vi "Test Graph Module API.vi"() -> ()   [LabVIEW 2020]
doc: "Graph Module API Tester."
uses:
  Graph Module.lvlib
panel:
  in  "X Backw":bool
  in  "Y Forw":bool
  in  "Y Backw":bool
  in  "X Forw":bool
  in  "XY Coord":cluster{"X":dbl, "Y":dbl}={"X"=1400.0, "Y"=200.0}
  in  "Mark Coord":bool
  in  "Path":path=path "D:/Git/Graph-Extensions-LabVIEW-master/dxf/#163_CAD2000_.dxf"
  in  "Load DXF":bool
  in  "Run as Singleton?":bool
  in  "Show Block Diagram":bool
  in  "Refresh Modules":bool
  out "Active Modules":string[](array[string])
  in  "Stop Module":bool
  in  "Select Module":i32(ring)=-1 caption="Select Module\nTo send Request to" items=["All"=-1, "1"=1]
  in  "Run New Module":bool
  in  "Hide Module Panel":bool
  in  "Show Module Panel":bool
  out "Status":string
  # "This VI tests the API for the Module."
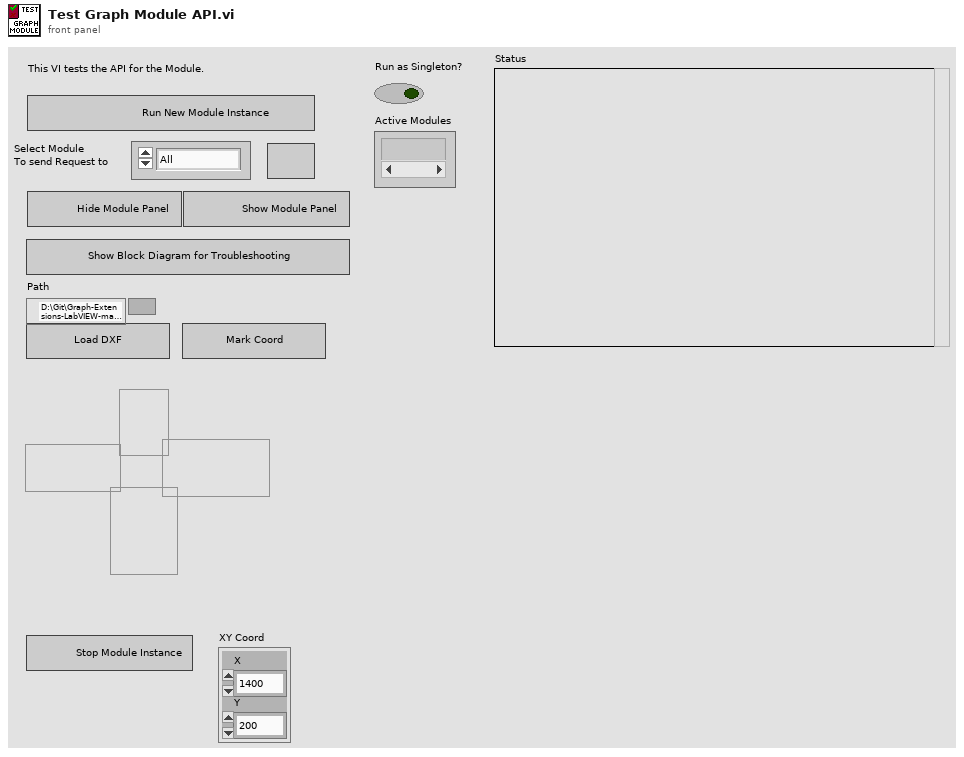
[diagram p1: front panel]
types:
  T1 = typedef "Graph Module.lvlib/Broadcast Events--cluster.ctl" = cluster{"Module Did Init":refnum<user-event>, "Status Updated":refnum<user-event>, "Error Reported":refnum<user-event>, "Module Did Stop":refnum<user-event>, "Update Module Execution Status":refnum<user-event>, "Broadcast Coord":refnum<user-event>}
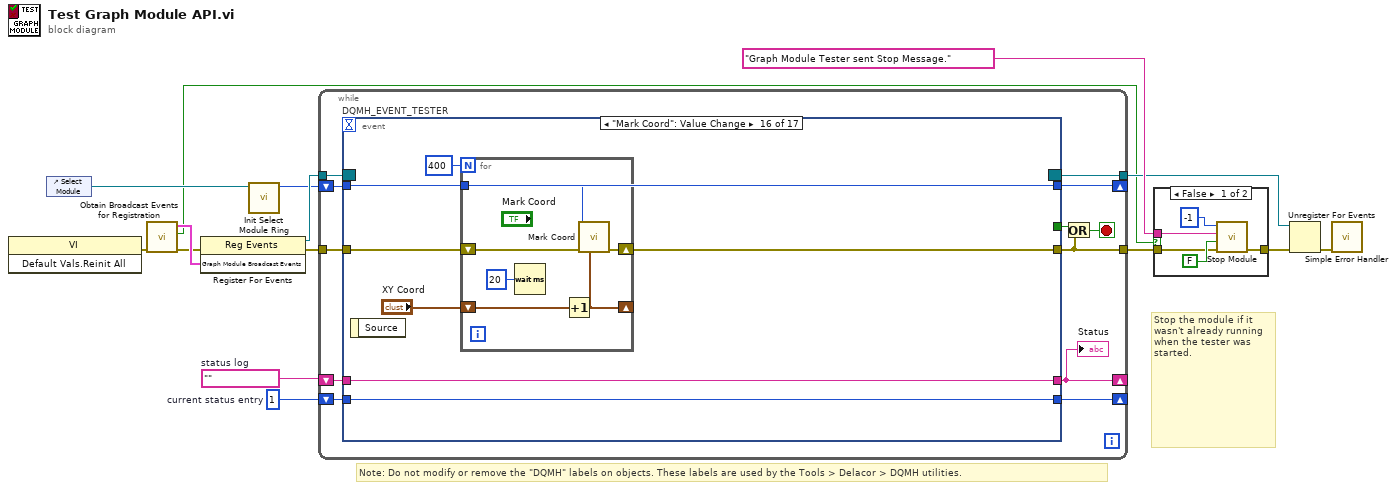
[diagram p0: block diagram]
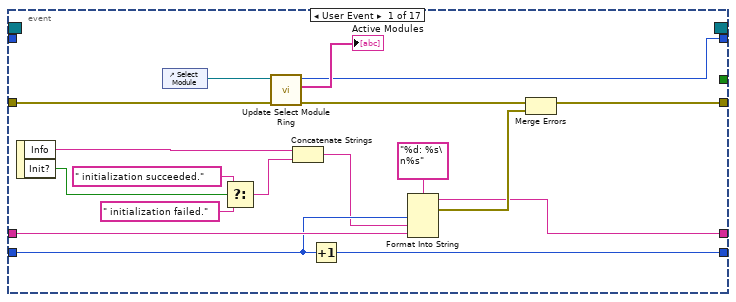
[diagram p3: hidden frame]
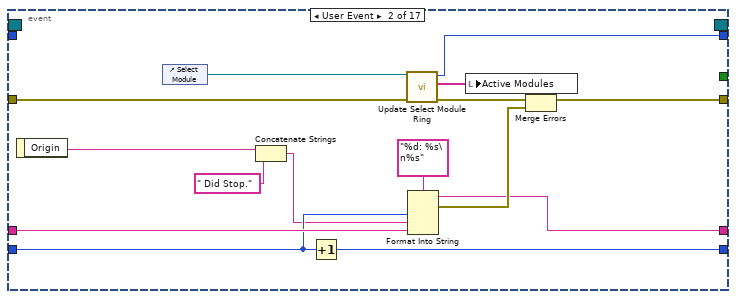
[diagram p4: hidden frame]
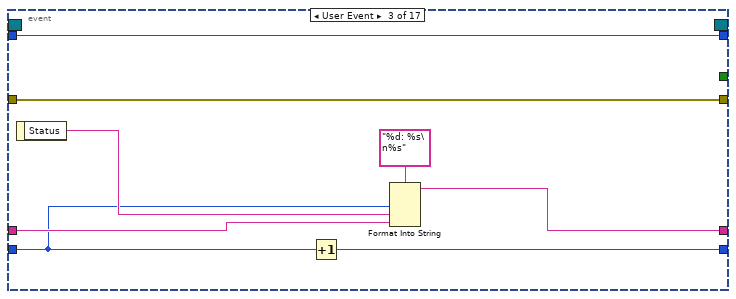
[diagram p5: hidden frame]
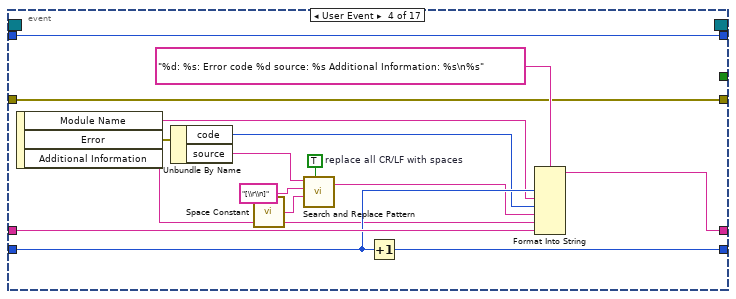
[diagram p6: hidden frame]
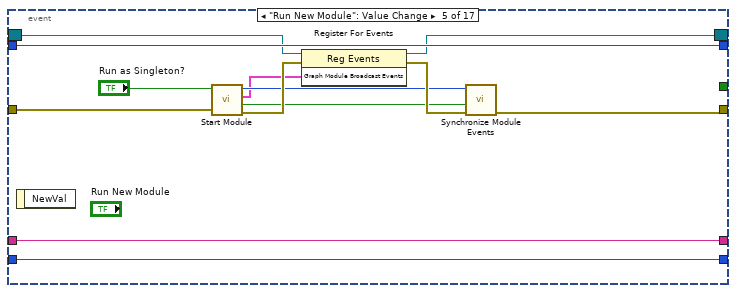
[diagram p7: hidden frame]
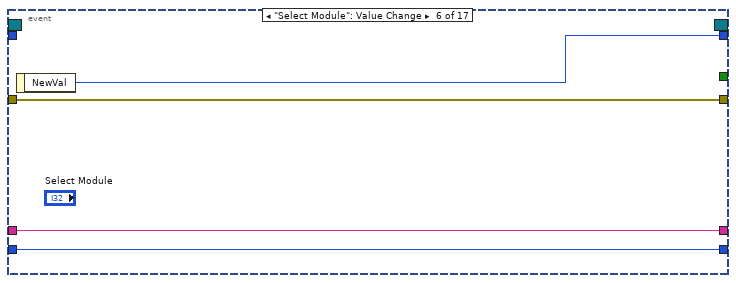
[diagram p8: hidden frame]
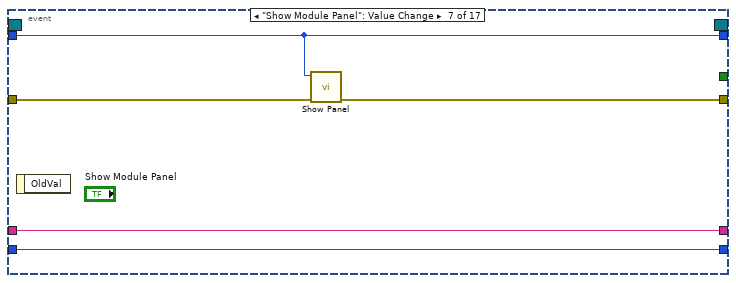
[diagram p9: hidden frame]
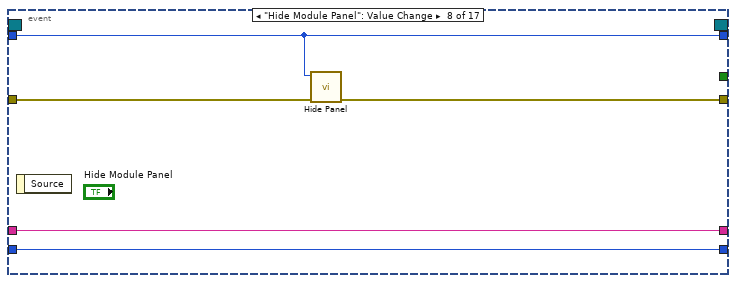
[diagram p10: hidden frame]
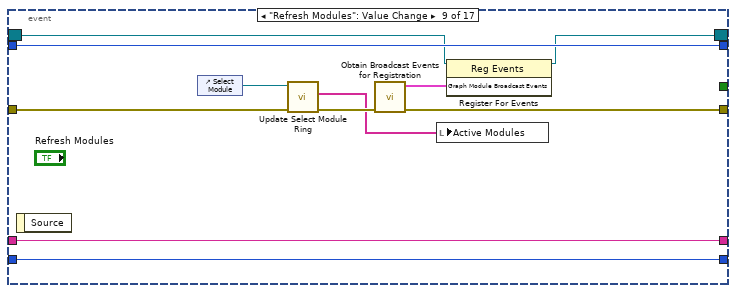
[diagram p11: hidden frame]
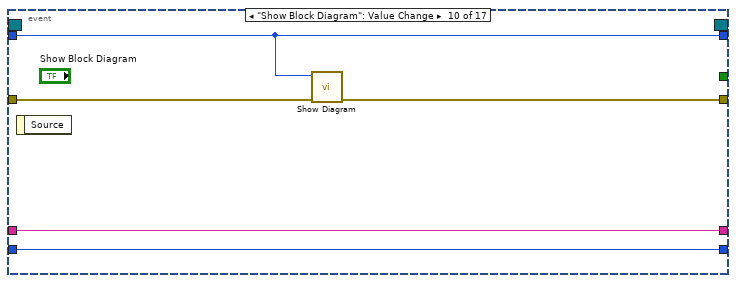
[diagram p12: hidden frame]
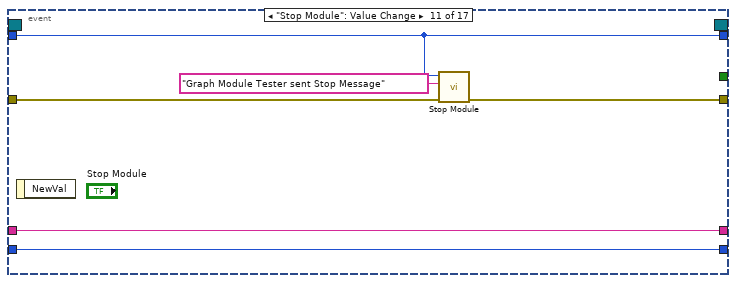
[diagram p13: hidden frame]
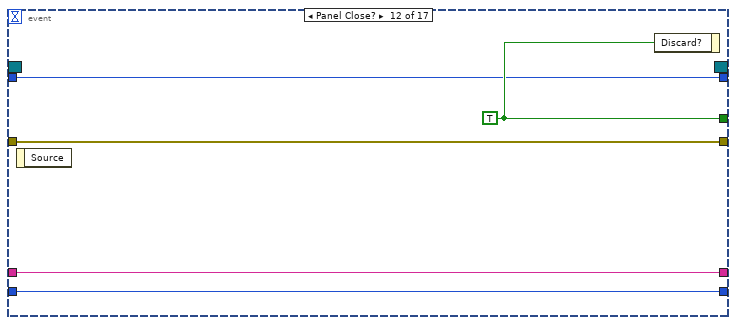
[diagram p14: hidden frame]
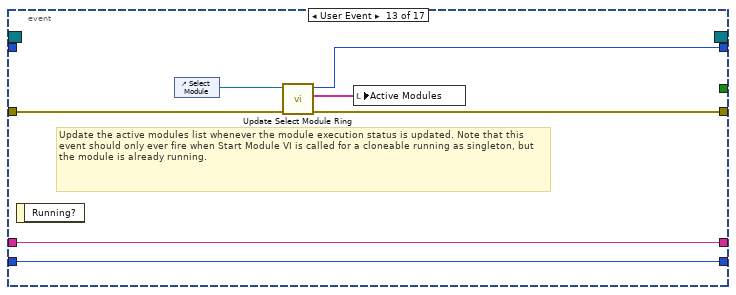
[diagram p15: hidden frame]
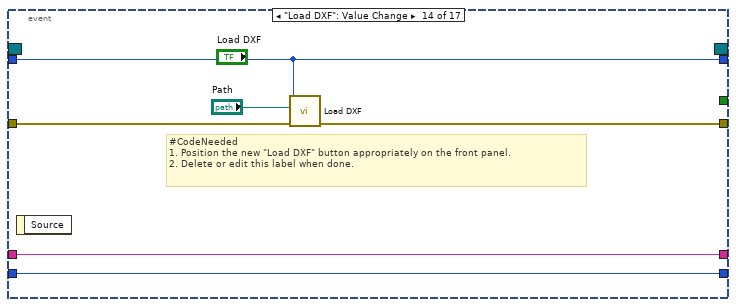
[diagram p16: hidden frame]
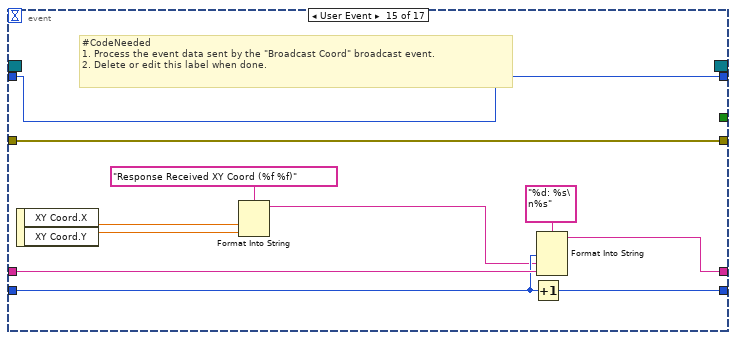
[diagram p17: hidden frame]
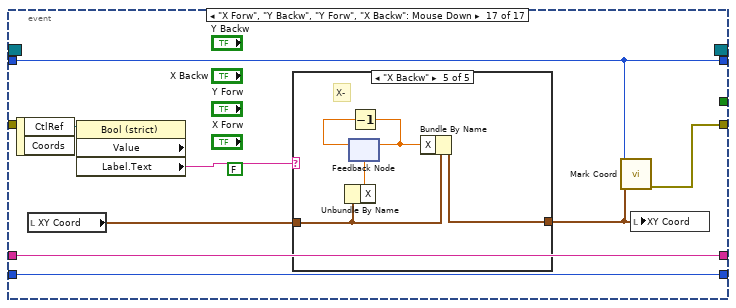
[diagram p18: hidden frame]
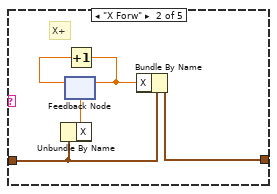
[diagram p20: hidden frame]
diagram:
  w12 = 1  # current status entry
  w13 = ""  # status log
  # "Stop the module if it wasn't already running when the tester was started."
  # "Note: Do not modify or remove the \"DQMH\" labels on objects. These labels are used by the Tools > Delacor > DQMH utilities."
  n1 = invoke class="VI" method="Default Vals.Reinit All"() -> (error out=w5:errorcluster)  [unwired: 3 in, 2 out]
  n2 = control-ref of="Select Module"() -> (w10:refnum<vi>)
  n3 = call "Obtain Broadcast Events for Registration.vi"("error in (no error)"=w5) -> ("error out"=w4:errorcluster, "Already running?"=w3:bool, "Graph Module Broadcast Events"=w9:T1)  [unwired: 8 in]
  n4 = register-events(error in=w4, w9) -> (reference out=w15:refnum<event-registration>, error out=w8:errorcluster)  [unwired: 1 in]
  n5 = call "Init Select Module Ring.vi"("Select Module Ring Ref"=w10) -> ("Value for All Modules"=w11:i32)  [unwired: 8 in, 2 out]
  n6 = while {
    tunnel: w15 -> [w27]
    tunnel: [w16] -> w2
    tunnel: w8 -> [w25]
    shift-right: [w21] -> _
    shift-left: w13 -> [w23]
    shift-right: [w22] -> _
    shift-left: w12 -> [w24]
    shift-right: [w18] -> _
    shift-left: w11 -> [w19]
    tunnel: [w17] -> w6
    stop <- w20 stop-if-true
    n7 = event "DQMH_EVENT_TESTER" shown="[15] \"Mark Coord\": Value Change" {
      selector: w27 -> [_ _ _ _ w91 _ _ _ w117 _ _ _ _ _ _ _ _]
      dyn-events: [_ _ _ _ w90 _ _ _ w116 _ _ _ _ _ _ _ _] -> w17
      timeout: _ -> [_ _ _ _ _ _ _ _ _ _ _ _ _ _ _ _ _]
      tunnel: [_ _ _ _ _ _ _ _ _ _ _ w138 _ _ _ _ _] -> w26
      tunnel: [w35 w52 w68 w74 w89 w101 w105 w110 w113 w124 w129 w137 w141 w148 w162 w166 w178] -> w16
      tunnel: w25 -> [w37 w54 w68 w74 w92 w101 w106 w111 w118 w127 w130 w137 w142 w151 w162 w169 _]
      tunnel: w24 -> [w42 w57 w61 w80 w94 w99 w103 w108 w121 w125 w132 w135 w144 w149 w158 w167 w182]
      tunnel: w23 -> [w43 w58 w64 w82 w95 w100 w104 w109 w122 w126 w133 w136 w145 w150 w160 w168 w183]
      tunnel: [w40 w55 w65 w77 w95 w100 w104 w109 w122 w126 w133 w136 w145 w150 w159 w168 w183] -> w21
      tunnel: [w41 w56 w67 w83 w94 w99 w103 w108 w121 w125 w132 w135 w144 w149 w157 w167 w182] -> w22
      tunnel: w19 -> [_ _ w62 w84 w93 _ w102 w107 w120 w123 w131 w134 _ w146 w161 w165 w179]
      tunnel: [w32 w49 w62 w84 w93 w98 w102 w107 w120 w123 w131 w134 w140 w146 w161 w165 w179] -> w18
      event User Event {
        n8 = event-data() -> ("Info"=w39:string, "Init?"=w29:bool)  [unwired: 1 in]
        n9 = control-ref of="Select Module"() -> (w34:refnum<vi>)
        n10 = Select(t=" initialization succeeded.", s=w29, f=" initialization failed.") -> (s? t:f=w28:string)
        n11 = call "Update Select Module Ring.vi"("error in (no error)"=w37, "Select Module Ring Ref"=w34) -> ("error out"=w36:errorcluster, "Active Modules (Array)"=→"Active Modules":string[], "New Module Ring Value"=w32:i32)  [unwired: 7 in]
        n12 = Concatenate Strings(w39, w28) -> (w38:string)
        n13 = Increment(x=w42) -> (x+1=w41:i32)
        n14 = Format Into String(format string="%d: %s\n%s", w42, w38, w43) -> (resulting string=w40:string, error out=w45:errorcluster)  [unwired: 2 in]
        n15 = Merge Errors(w36, w45) -> (w35:errorcluster)
      }
      event User Event {
        n16 = event-data() -> ("Origin"=w47:string)  [unwired: 1 in]
        n17 = control-ref of="Select Module"() -> (w51:refnum<vi>)
        n18 = Concatenate Strings(w47, " Did Stop.") -> (w46:string)
        n19 = Increment(x=w57) -> (x+1=w56:i32)
        n20 = call "Update Select Module Ring.vi"("error in (no error)"=w54, "Select Module Ring Ref"=w51) -> ("error out"=w53:errorcluster, "Active Modules (Array)"=w50:string[], "New Module Ring Value"=w49:i32)  [unwired: 7 in]
        n21 = Format Into String(format string="%d: %s\n%s", w57, w46, w58) -> (resulting string=w55:string, error out=w60:errorcluster)  [unwired: 2 in]
        n22 = local write "Active Modules"(w50) -> ()
        n23 = Merge Errors(w53, w60) -> (w52:errorcluster)
      }
      event User Event {
        n24 = event-data() -> ("Status"=w63:string)  [unwired: 1 in]
        n25 = Increment(x=w61) -> (x+1=w67:i32)
        n26 = Format Into String(format string="%d: %s\n%s", w61, w63, w64) -> (resulting string=w65:string)  [unwired: 2 in, 1 out]
      }
      event User Event {
        w78 = TRUE  # replace all CR/LF with spaces
        n27 = event-data() -> ("Module Name"=w72:string, "Error"=w71:errorcluster, "Additional Information"=w69:string)  [unwired: 1 in]
        n28 = Unbundle By Name(w71) -> ("code"=w73:i32, "source"=w75:string)
        n29 = call <vilib>:"Space Constant.vi"() -> ("String"=w79:string)
        n30 = call <vilib>:"Search and Replace Pattern.vi"("string"=w75, "regular expression (\"\")"="[\\r\\n]" ("regular expression (\"\")"), "replace string (\"\")"=w79, "replace all? (F)"=w78) -> ("result string"=w76:string)  [unwired: 1 in, 1 out]
        n31 = Increment(x=w80) -> (x+1=w83:i32)
        n32 = Format Into String(format string="%d: %s: Error code %d source: %s Additional Information: %s\n%s", w80, w72, w73, w76, w69, w82) -> (resulting string=w77:string)  [unwired: 2 in, 1 out]
      }
      event "Run New Module": Value Change {
        n33 = event-data() -> ()  [unwired: 1 in, 1 out]
        n34 = call "Start Module.vi"("error in"=w92, "Run as Singleton? (F)"="Run as Singleton?") -> ("error out"=w96:errorcluster, "Wait for Event Sync?"=w87:bool, "Graph Module Broadcast Events"=w86:T1, "Module ID"=w88:i32)  [unwired: 6 in]
        n35 = register-events(reference=w91, error in=w96, w86) -> (reference out=w90:refnum<event-registration>, error out=w97:errorcluster)
        n36 = call "Synchronize Module Events.vi"("error in"=w97, "Wait for Event Sync?"=w87, "Module ID in"=w88) -> ("error out"=w89:errorcluster)  [unwired: 7 in, 1 out]
      }
      event "Select Module": Value Change {
        n37 = event-data() -> ("NewVal"=w98:i32)  [unwired: 1 in]
      }
      event "Show Module Panel": Value Change {
        n38 = event-data() -> ()  [unwired: 1 in, 1 out]
        n39 = call "Show Panel.vi"("error in (no error)"=w106, "Module ID"=w102) -> ("error out"=w105:errorcluster)  [unwired: 9 in]
      }
      event "Hide Module Panel": Value Change {
        n40 = event-data() -> ()  [unwired: 1 in, 1 out]
        n41 = call "Hide Panel.vi"("error in (no error)"=w111, "Module ID"=w107) -> ("error out"=w110:errorcluster)  [unwired: 9 in]
      }
      event "Refresh Modules": Value Change {
        n42 = event-data() -> ()  [unwired: 1 in, 1 out]
        n43 = control-ref of="Select Module"() -> (w119:refnum<vi>)
        n44 = call "Update Select Module Ring.vi"("error in (no error)"=w118, "Select Module Ring Ref"=w119) -> ("error out"=w114:errorcluster, "Active Modules (Array)"=w112:string[])  [unwired: 7 in, 1 out]
        n45 = call "Obtain Broadcast Events for Registration.vi"("error in (no error)"=w114) -> ("error out"=w113:errorcluster, "Graph Module Broadcast Events"=w115:T1)  [unwired: 8 in, 1 out]
        n46 = local write "Active Modules"(w112) -> ()
        n47 = register-events(reference=w117, w115) -> (reference out=w116:refnum<event-registration>)  [unwired: 1 in, 1 out]
      }
      event "Show Block Diagram": Value Change {
        n48 = event-data() -> ()  [unwired: 1 in, 1 out]
        n49 = call "Show Diagram.vi"("error in (no error)"=w127, "Module ID"=w123) -> ("error out"=w124:errorcluster)  [unwired: 9 in]
      }
      event "Stop Module": Value Change {
        n50 = event-data() -> ()  [unwired: 1 in, 1 out]
        n51 = call "Stop Module.vi"("error in (no error)"=w130, "Origin"="Graph Module Tester sent Stop Message", "Module ID"=w131) -> ("error out"=w129:errorcluster)  [unwired: 8 in]
      }
      event Panel Close? {
        w138 = TRUE ("Discard?")
        n52 = event-data() -> ()  [unwired: 1 in, 1 out]
        n53 = event-data("Discard?"=w138) -> ()  [unwired: 1 in, 1 out]
      }
      event User Event {
        # "Update the active modules list whenever the module execution status is updated. Note that this event should only ever fire when Start Module VI is called for a cloneable running as singleton, but the module is already running."
        n54 = event-data() -> ()  [unwired: 1 in, 1 out]
        n55 = control-ref of="Select Module"() -> (w143:refnum<vi>)
        n56 = call "Update Select Module Ring.vi"("error in (no error)"=w142, "Select Module Ring Ref"=w143) -> ("error out"=w141:errorcluster, "Active Modules (Array)"=w139:string[], "New Module Ring Value"=w140:i32)  [unwired: 7 in]
        n57 = local write "Active Modules"(w139) -> ()
      }
      event "Load DXF": Value Change {
        # "#CodeNeeded\n1. Position the new \"Load DXF\" button appropriately on the front panel.\n2. Delete or edit this label when done."
        n58 = event-data() -> ()  [unwired: 1 in, 1 out]
        n59 = call "Load DXF.vi"("error in"=w151, "Path"="Path", "Module ID"=w146) -> ("error out"=w148:errorcluster)  [unwired: 8 in]
      }
      event User Event {
        # "#CodeNeeded\n1. Process the event data sent by the \"Broadcast Coord\" broadcast event.\n2. Delete or edit this label when done."
        n60 = event-data() -> ("XY Coord.X"=w153:dbl, "XY Coord.Y"=w152:dbl)  [unwired: 1 in]
        n61 = Format Into String(format string="Response Received XY Coord (%f %f)", w153, w152) -> (resulting string=w154:string)  [unwired: 2 in, 1 out]
        n62 = Increment(x=w158) -> (x+1=w157:i32)
        n63 = Format Into String(format string="%d: %s\n%s", w158, w154, w160) -> (resulting string=w159:string)  [unwired: 2 in, 1 out]
      }
      event "Mark Coord": Value Change {
        n64 = event-data() -> ()  [unwired: 1 in, 1 out]
        n65 = for {
          N: 400 -> [_]
          tunnel: w165 -> [w173]
          shift-right: [w174] -> w166
          shift-left: w169 -> [w175]
          shift-right: [w170] -> _
          shift-left: "XY Coord" -> [w172]
          n66 = Wait (ms)(milliseconds to wait=u32 20) -> ()  [unwired: 1 out]
          n67 = Increment(x=w172) -> (x+1=w170:cluster{"X":dbl, "Y":dbl})
          n68 = call "Mark Coord.vi"("error in"=w175, "XY Coord"=w170, "Module ID"=w173) -> ("error out"=w174:errorcluster)  [unwired: 8 in]
        }
      }
      event "X Forw", "Y Backw", "Y Forw", "X Backw": Mouse Down {
        (unwired) FALSE
        n69 = event-data() -> ("CtlRef"=w176:refnum<vi>)  [unwired: 1 in, 1 out]
        n70 = local read "XY Coord"() -> (w181:cluster{"X":dbl, "Y":dbl})
        n71 = property class="Bool (strict)" props=["Value", "Label", "Text"](reference=w176) -> ("Label.Text"=w177:string)  [unwired: 1 in, 3 out]
        n72 = case shown="\"X Backw\"" w177 {
          tunnel: w181 -> [w184 w187 w192 w197 w202]
          tunnel: [w184 w185 w190 w195 w200] -> w180
          frame "0", Default {
          }
          frame "X Forw" {
            # "X+"
            n73 = Unbundle By Name(w187) -> ("X"=w186:dbl)
            n74 = feedback #1(w186) -> (w188:dbl)
            n75 = Increment(x=w188) -> (x+1=w189:dbl)
            n76 = feedback-in #1(w189) -> ()
            n77 = Bundle By Name(cluster=w187, "X"=w189) -> (w185:cluster{"X":dbl, "Y":dbl})
          }
          frame "Y Backw" {
            # "Y-"
            n78 = Unbundle By Name(w192) -> ("Y"=w191:dbl)
            n79 = feedback #2(w191) -> (w193:dbl)
            n80 = Decrement(x=w193) -> (x-1=w194:dbl)
            n81 = feedback-in #2(w194) -> ()
            n82 = Bundle By Name(cluster=w192, "Y"=w194) -> (w190:cluster{"X":dbl, "Y":dbl})
          }
          frame "Y Forw" {
            # "Y+"
            n83 = Unbundle By Name(w197) -> ("Y"=w196:dbl)
            n84 = feedback #3(w196) -> (w198:dbl)
            n85 = Increment(x=w198) -> (x+1=w199:dbl)
            n86 = feedback-in #3(w199) -> ()
            n87 = Bundle By Name(cluster=w197, "Y"=w199) -> (w195:cluster{"X":dbl, "Y":dbl})
          }
          frame "X Backw" {
            # "X-"
            n88 = Unbundle By Name(w202) -> ("X"=w201:dbl)
            n89 = feedback #4(w201) -> (w203:dbl)
            n90 = Decrement(x=w203) -> (x-1=w204:dbl)
            n91 = feedback-in #4(w204) -> ()
            n92 = Bundle By Name(cluster=w202, "X"=w204) -> (w200:cluster{"X":dbl, "Y":dbl})
          }
        }
        n93 = call "Mark Coord.vi"("XY Coord"=w180, "Module ID"=w179) -> ("error out"=w178:errorcluster)  [unwired: 9 in]
        n94 = local write "XY Coord"(w180) -> ()
      }
    }
    "Status" <- w21
    n95 = Or(x=w26, y=w16) -> (x .or. y?=w20:bool)
  }
  n96 = case shown="False" w3 {
    tunnel: [w209 w210] -> w14
    tunnel: "Graph Module Tester sent Stop Message." ("Origin") -> [w208 _]
    tunnel: w2 -> [w205 w210]
    frame False {
      n97 = call "Stop Module.vi"("error in (no error)"=w205, "Wait for Module to stop? (F)"=FALSE ("Wait for Module to stop?"), "Origin"=w208, "Module ID"=-1 ("Stop all")) -> ("error out"=w209:errorcluster)  [unwired: 7 in]
    }
    frame True {
    }
  }
  n98 = Unregister For Events(event registration refnum=w6, error in=w14) -> (error out=w1:errorcluster)
  n99 = call <vilib>:"Simple Error Handler.vi"("error in (no error)"=w1) -> ()  [unwired: 4 in, 5 out]
